vi "jt_data_to_plot.vi"(8 "Data Array 2":dbl[][](array[numeric]), 11 "Data Array":dbl[][](array[numeric])) -> (3 "JV Curve":cluster{"Y":dbl[], "Y":dbl[]}[](graph))   [LabVIEW 2016]
panel:
  in  "Tab Control 4":enum32{"Page 1"}(tab)
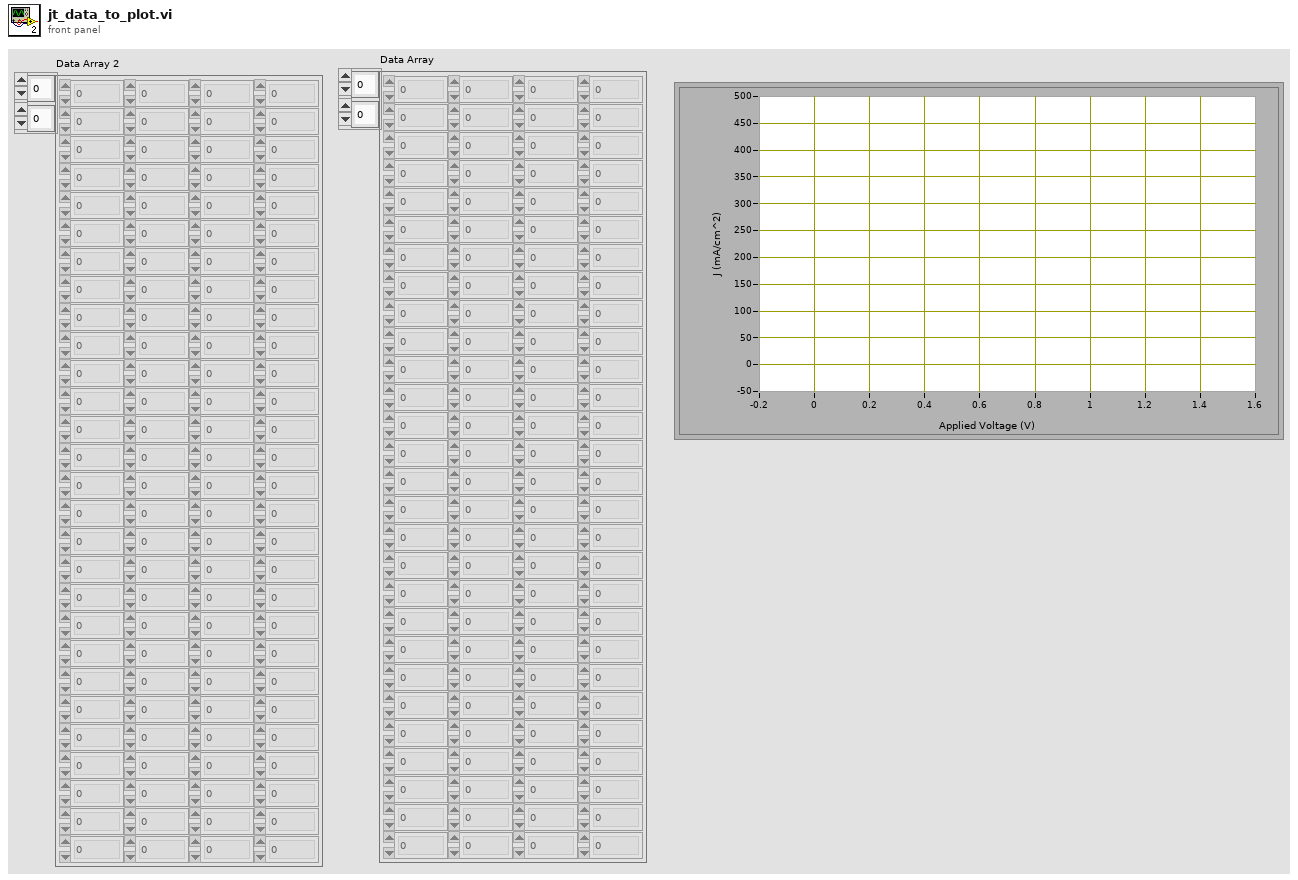
[diagram p1: front panel]
types:
  T1 = cluster{"Data Array 2":dbl[], "Data Array 2":dbl[]}
  T2 = cluster{"Data Array 2":dbl[], "Data Array 2":dbl[]}[]
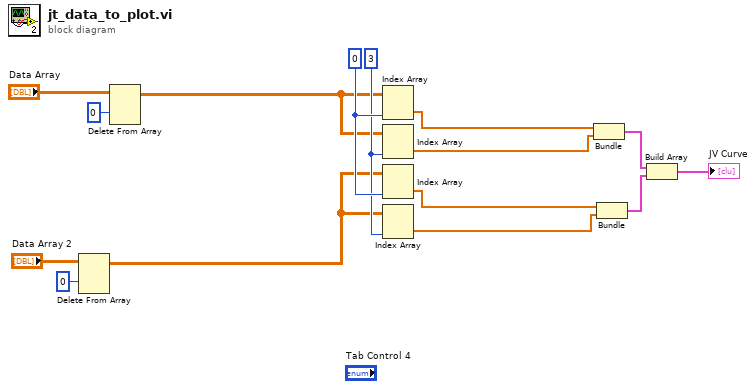
[diagram p0: block diagram]
diagram:
  w3 = 3
  w4 = 0
  n1 = Delete From Array(array="Data Array 2", index (row)=0) -> (array with subset deleted=w1:dbl[][])  [unwired: 2 in, 1 out]
  n2 = Delete From Array(array="Data Array", index (row)=0) -> (array with subset deleted=w2:dbl[][])  [unwired: 2 in, 1 out]
  n3 = Index Array(array=w2, index (col)=w4) -> (element=w15:dbl[])  [unwired: 1 in]
  n4 = Index Array(array=w2, index (col)=w3) -> (element=w10:dbl[])  [unwired: 1 in]
  n5 = Index Array(array=w1, index (col)=w4) -> (element=w14:dbl[])  [unwired: 1 in]
  n6 = Index Array(array=w1, index (col)=w3) -> (element=w9:dbl[])  [unwired: 1 in]
  n7 = Bundle("Data Array"=w15, "Data Array"=w10) -> (w12:cluster{"Data Array":dbl[], "Data Array":dbl[]})  [unwired: 1 in]
  n8 = Bundle("Data Array 2"=w14, "Data Array 2"=w9) -> (w13:T1)  [unwired: 1 in]
  n9 = Build Array(w12, w13) -> (→"JV Curve":T2)
